vi "题目三.vi"() -> ()   [LabVIEW 2017]
panel:
  out "数组":dbl[][](array[numeric])
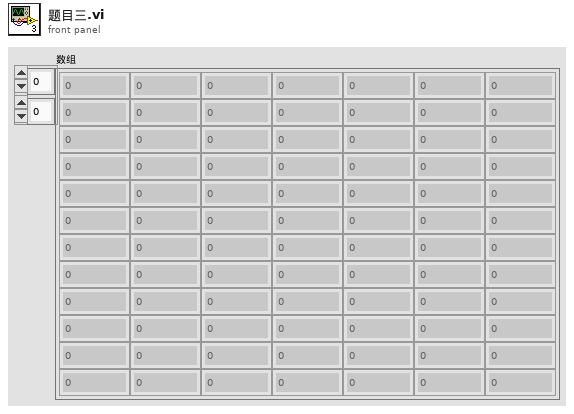
[diagram p1: front panel]
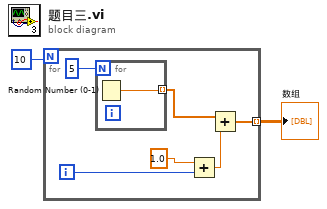
[diagram p0: block diagram]
diagram:
  n1 = for {
    N: 10 -> [_]
    tunnel: [w6] -> w1 mode=indexing
    i -> [w4]
    n2 = for {
      N: 5 -> [_]
      tunnel: [w9] -> w7 mode=indexing
      n3 = Random Number (0-1)() -> (number: 0 to 1=w9:dbl)
    }
    n4 = Add(x=1.0, y=w4) -> (x+y=w3:dbl)
    n5 = Add(x=w7, y=w3) -> (x+y=w6:dbl[])
  }
  "数组" <- w1
